vi "Dashboard Main.vi"() -> ()   [LabVIEW 2013]
uses:
  <vilib>/event_ctls.llb/eventvkey.ctl
  <vilib>/Rock Robotics/WPI/Dashboard/WPI_DashboardLogging Global.vi
  <vilib>/Utility/config.llb/Write Key (String).vi
  <vilib>/Utility/config.llb/Write Key (I32).vi
  <vilib>/Utility/config.llb/NI_LVConfig.lvlib
panel:
  in  "Camera Settings":T1={"Frame Rate"=30, "Compression"=30, "Size"=1} {"Frame Rate" scale=1.0..30.0; "Size" items=["640x480", "320x240", "160x120"]}
  out "fps":dbl format="%#.1g"
  out "Mbps":dbl format="%#.1g"
  out "Mbps 2":bool
  in  "DB Camera Config":bool
  out "Image Message":string="Timeout in Camera Communications"
  in  "Rec Mode":enum32{"Stop", "Record", "Playback"}(radio)
  in  "Dashboard Tab":T2(tab)
  out "Robot Mode":dbl
  out "Motor Current":dbl[](array[numeric])
  out "Compressor Relay Status":bool
  out "Compressor Control Status":bool
  in  "Compressor Control":bool
  in  "Jag Position Enable":bool
  out "Right Direction Motor Position":dbl
  out "Left Direction Motor Position":dbl
  out "MotorSliders R":cluster{"MotorSlide1":dbl, "MotorSlide2":dbl} {"MotorSlide2" scale=-1.0..1.0 scale format="%#_2e"; "MotorSlide1" scale=-1.0..1.0 scale format="%#_2e"}
  out "MotorChart R":cluster{"Numeric":dbl, "Numeric":dbl}(graph)
  out "MotorSliders L":T3 {"MotorSlide4 2" scale=0.0..14.0 scale format="%#_2e"; "MotorSlide2" scale=-1.0..1.0 scale format="%#_2e"; "MotorSlide1" scale=-1.0..1.0 scale format="%#_2e"}
  out "MotorChart L":T4(graph)
  out "JS1 Z":dbl(slide) scale=-1.0..1.0 scale format="%#_2e"
  out "Joystick 1":cluster{"X":dbl, "Y":dbl}[](graph)
  out "JS Buttons 1":T5
  out "JS2 Z":dbl(slide) scale=-1.0..1.0 scale format="%#_2e"
  out "Joystick 2":cluster{"X":dbl, "Y":dbl}[](graph)
  out "JS Buttons 2":T5
  out "Mode":T6(ring)=enum."Auto Disabled"
  out "Camera IP":string
  out "Jag 6":dbl(graph)
  out "Jag 1":dbl(graph)
  out "Jag 8":dbl(graph)
  out "Jag 3":dbl(graph)
  in  "Test Slider":dbl(slide) scale=0.0..100.0 scale format="%#_3g"
  in  "On/Off":bool caption="Solenoid"
  in  "Test Name":u16(ring) items=["Select the test to run..."]
  in  "Test Tree":string(tree)
  in  "Motor":cluster{"Value":dbl, "Enable":bool} {"Value" scale=-1.0..1.0 scale format="%#_3g"}
  out "Progress":T7 {"Test Progress" scale=0.0..100.0}
  in  "Rev/Fwd":cluster{"Forward":bool, "Reverse":bool}
  in  "Test Ring":u16(ring) items=["Auto", "Fixed indoor", "Fixed outdoor 1", "Fixed outdoor 2", "Fixed fluorescent 1", "Fixed fluorescent 2", "Hold current"]
  in  "Listbox":i32(listbox)
  out "Tree":string(tree)
  out "Camera Image":T8(plugin-control)
  in  "Enable":bool
  # "Left"
  # "Right"
  # "Battery"
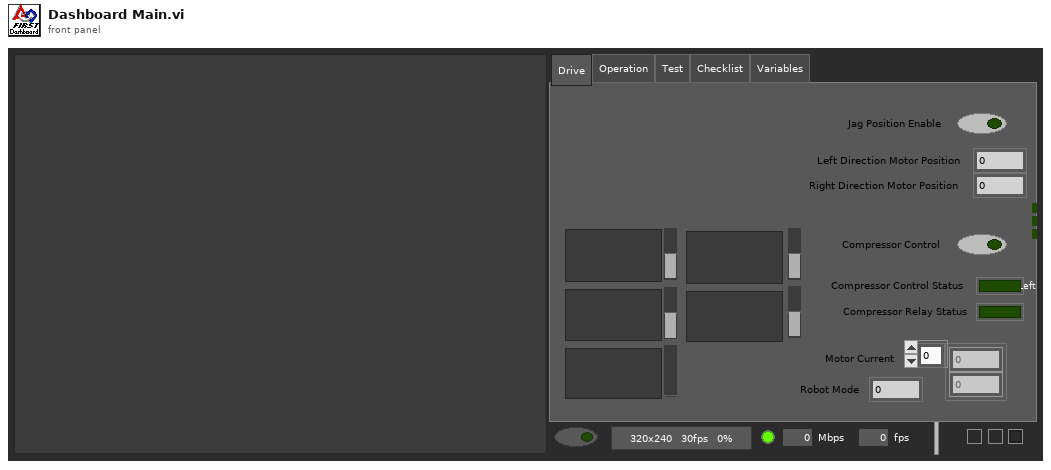
[diagram p1: front panel]
types:
  T1 = cluster{"Frame Rate":i32, "Compression":i32, "Size":u16}
  T2 = enum32{"Drive", "Operation", "Test", "Checklist", "Variables"}
  T3 = cluster{"MotorSlide1":dbl, "MotorSlide2":dbl, "MotorSlide4 2":dbl}
  T4 = cluster{"Numeric":dbl, "Numeric":dbl, "Battery":sgl}
  T5 = cluster{bool, bool, bool, bool, bool, bool, bool, bool, bool, bool, bool, bool}
  T6 = enum8{"Tele-Op Disabled", "Tele-Op Enabled", "Auto Disabled", "Auto Enabled", "Test Disabled", "Test Enabled", ""}
  T7 = cluster{"Test Progress":u8, "Test Progress Text":string}
  T8 = typedef "IMAQ Image.ctl" = refnum<image>
  T9 = enum32{"Drive", "Operation", "Auto", "Test", "Checklist", "Variables"}
  T10 = typedef "Image Type" = u32
  T11 = cluster{"Digital Inputs":bool[], "Digital Outputs":bool[]}
  T12 = cluster{"Competition mode":bool, "Robot Link":bool, "Autonomous":bool, "Enabled":bool, "E-Stop":bool, "Simulated":bool, "TestMode":bool, "Docked Window":bool}
  T13 = cluster{"Boolean Array[0]":bool, "Boolean Array[1]":bool, "Boolean Array[2]":bool, "Boolean Array[3]":bool, "Boolean Array[4]":bool, "Boolean Array[5]":bool, "Boolean Array[6]":bool, "Boolean Array[7]":bool, "Boolean Array[8]":bool, "Boolean Array[9]":bool, "Boolean Array[10]":bool, "Boolean Array[11]":bool}
  T14 = typedef "NI_LVConfig.lvlib/Config Data RefNum.ctl" = refnum<k1>
  T15 = typedef "eventvkey.ctl" = enum16{"ASCII", "Enter", "Return", "Shift", "Ctrl", "Alt", "Cmd", "Opt", "Caps", "NumLock", "Clear", "Break", "Up", "Down", "Left", "Right", "Insert", "Delete", "Home", "End", "PageUp", "PageDown", "Escape", "Help", "Pause", "ScrollLock", "F1", "F2", "F3", "F4", "F5", "F6", "F7", "F8", "F9", "F10", "F11", "F12", "F13", "F14", "F15", "F16", "F17", "F18", "F19", "F20", "F21", "F22", "F23", "F24", "Play", "VolumeUp", "VolumeDown", "Mute", "Two Byte Char"}
  T16 = cluster{"Image Size":bool, "Image Type":bool, "Pixel Value":bool, "ROI Information":bool, "Zoom Factor":bool}
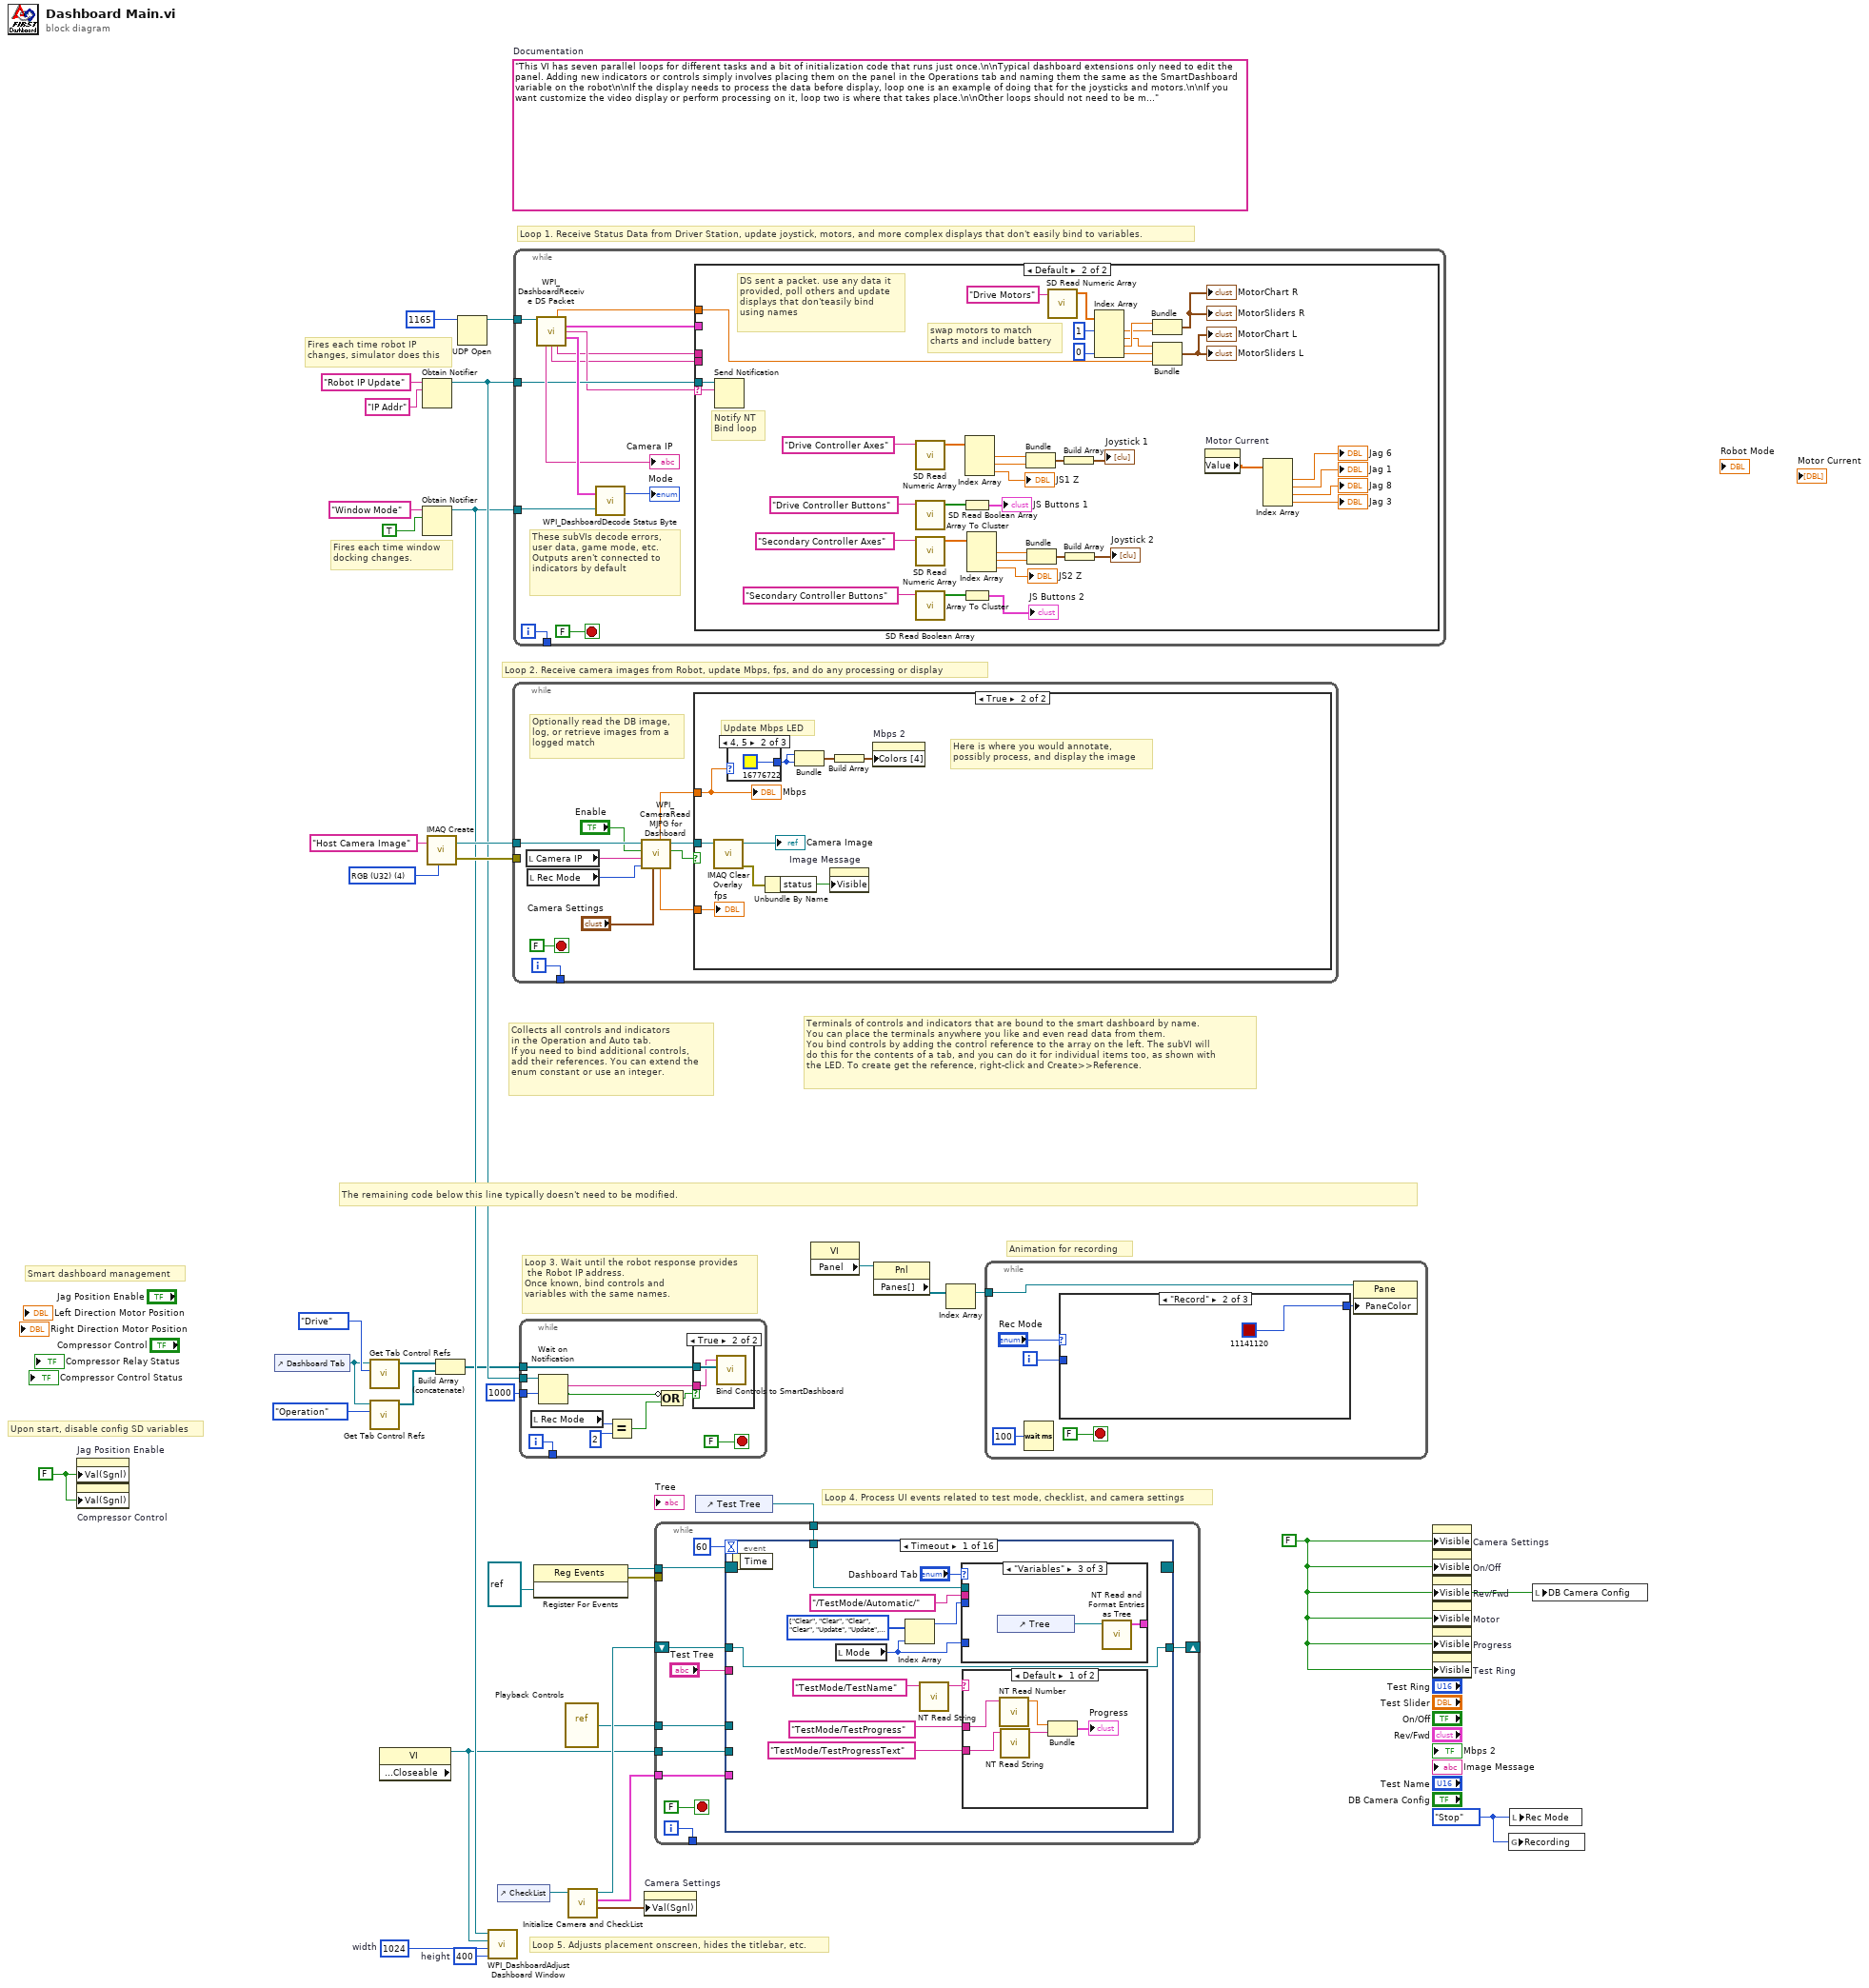
[diagram p0: block diagram]
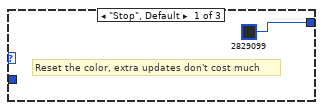
[diagram p2: hidden frame]
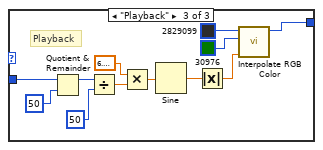
[diagram p3: hidden frame]
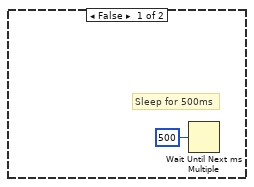
[diagram p5: hidden frame]
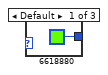
[diagram p6: hidden frame]
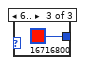
[diagram p7: hidden frame]
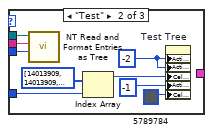
[diagram p9: hidden frame]
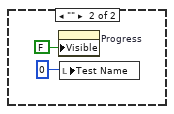
[diagram p10: hidden frame]
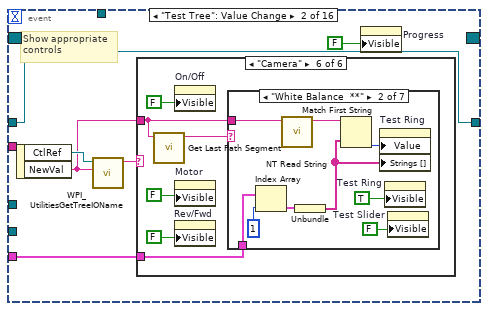
[diagram p11: hidden frame]
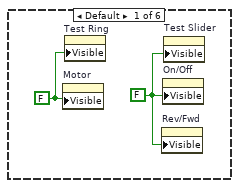
[diagram p12: hidden frame]
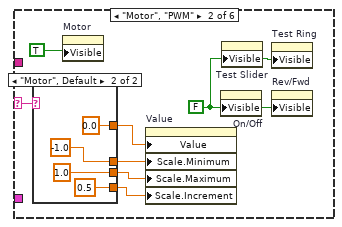
[diagram p13: hidden frame]
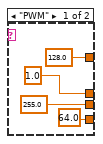
[diagram p14: hidden frame]
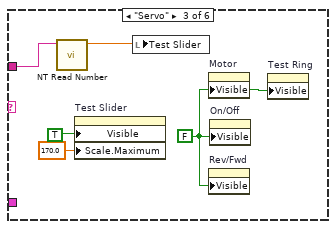
[diagram p15: hidden frame]
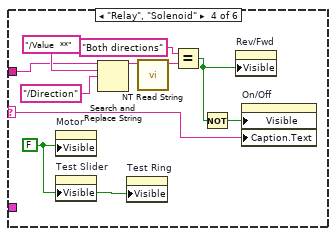
[diagram p16: hidden frame]
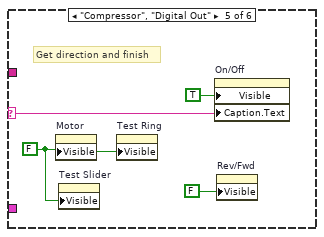
[diagram p17: hidden frame]
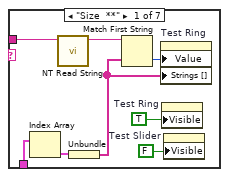
[diagram p18: hidden frame]
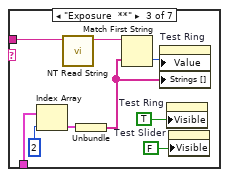
[diagram p19: hidden frame]
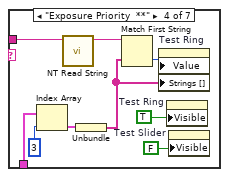
[diagram p20: hidden frame]
diagram:
  w1 = FALSE ("Value (Signaling)")
  w8 = enum32{"Stop", "Record", "Playback"}."Stop" ("Rec Mode")
  w11 = 400  # height
  w12 = 1024  # width
  w25 = FALSE ("Visible")
  (unwired) "This VI has seven parallel loops for different tasks and a bit of initialization code that runs just once.\n\nTypical dashboard extensions only need to edit the panel. Adding new indicators or controls simply involves placing them on the panel in the Operations tab and naming them the same as the SmartDashboard variable on the robot\n\nIf the display needs to process the data before display, loop one is an example of doing that for the joysticks and motors.\n\nIf you want customize the video display or perform processing on it, loop two is where that takes place.\n\nOther loops should not need to be modified. They are pretty standard, and document the task they perform."  # Documentation
  w35 = T10 4 items=["Grayscale (U8)", "Grayscale (I16)", "Grayscale (SGL)", "Complex (CSG)", "RGB (U32)", "HSL (U32)", "RGB (U64)"] ("Image Type")
  # "Upon start, disable config SD variables"
  # "Smart dashboard management"
  # "Animation for recording"
  # "Fires each time robot IP\nchanges, simulator does this"
  # "Fires each time window\ndocking changes."
  # "Collects all controls and indicators\nin the Operation and Auto tab.\nIf you need to bind additional controls,\nadd their references. You can extend the\nenum constant or use an integer."
  # "The remaining code below this line typically doesn't need to be modified."
  # "Loop 4. Process UI events related to test mode, checklist, and camera settings"
  # "Terminals of controls and indicators that are bound to the smart dashboard by name.\nYou can place the terminals anywhere you like and even read data from them.\nYou bind controls by adding the control reference to the array on the left. The subVI will\ndo this for the contents of a tab, and you can do it for individual items too, as shown with\nthe LED. To create get the reference, right-click and Create>>Reference."
  # "Loop 3. Wait until the robot response provides\n the Robot IP address.\nOnce known, bind controls and\nvariables with the same names."
  # "Loop 5. Adjusts placement onscreen, hides the titlebar, etc."
  # "Loop 1. Receive Status Data from Driver Station, update joystick, motors, and more complex displays that don't easily bind to variables."
  # "Loop 2. Receive camera images from Robot, update Mbps, fps, and do any processing or display"
  n1 = property on="Jag Position Enable" class="Bool (strict)"("Val(Sgnl)"=w1) -> ()  [unwired: 2 in, 2 out]
  n2 = property on="Compressor Control" class="Bool (strict)"("Val(Sgnl)"=w1) -> ()  [unwired: 2 in, 2 out]
  n3 = control-ref of="Dashboard Tab"() -> (w6:refnum<vi>)
  n4 = call <vilib>:"Get Tab Control Refs.vi"("Page Index"=T9."Drive" ("Dashboard Tab"), "TabControl in"=w6) -> ("ControlsOnPage"=w4:refnum<vi>[])  [unwired: 9 in]
  n5 = call <vilib>:"Get Tab Control Refs.vi"("Page Index"=T9."Operation" ("Dashboard Tab"), "TabControl in"=w6) -> ("ControlsOnPage"=w5:refnum<vi>[])  [unwired: 9 in]
  n6 = property class="VI" props=["Front Panel.Closeable"]() -> (reference out=w7:refnum<vi>)  [unwired: 2 in, 2 out]
  n7 = Obtain Notifier(name (unnamed)="Robot IP Update", notification data type="IP Addr" ("name (unnamed)")) -> (notifier out=w29:refnum<notifier>)  [unwired: 2 in, 2 out]
  n8 = Obtain Notifier(name (unnamed)="Window Mode", notification data type=TRUE) -> (notifier out=w10:refnum<notifier>)  [unwired: 2 in, 2 out]
  n9 = call "IMAQ Create"("Image Name"="Host Camera Image", "Image Type"=w35) -> ("New Image"=w33:T8, "error out"=w32:errorcluster)  [unwired: 2 in, 1 out]
  n10 = Build Array (concatenate)(w4, w5) -> (w3:refnum<vi>[])
  n11 = UDP Open(11:u16 1165 ("port")) -> (port=w36:refnum<k16>)  [unwired: 2 in, 4 out]
  n12 = call <vilib>:"WPI_DashboardAdjust Dashboard Window.vi"("height"=w11, "width"=w12, "reference in"=w7, "Notifier in"=w10) -> ()  [unwired: 8 in]
  n13 = control-ref of="CheckList"() -> (w9:refnum<vi>)
  n14 = while {
    tunnel: w33 -> [w46]
    tunnel: w32 -> [_]
    tunnel: [w47] -> _
    i -> [w47]
    stop <- FALSE stop-if-true
    # "Optionally read the DB image,\nlog, or retrieve images from a\nlogged match"
    n15 = local read "Camera IP"() -> (w39:string)
    n16 = local read "Rec Mode"() -> (w38:enum32{"Stop", "Record", "Playback"})
    n17 = call <vilib>:"WPI_CameraRead MJPG for Dashboard.vi"("Camera Settings"="Camera Settings", "Rec Mode"=w38, "Camera IP"=w39, "Enable"="Enable", "Refnum in"=w46) -> ("Active"=w43:bool, "Refnum out"=w45:T8, "FPS"=w42:dbl, "Bandwidth (Mbps)"=w41:dbl)  [unwired: 3 in]
    n18 = case shown="True" w43 {
      tunnel: w45 -> [_ w53]
      tunnel: w41 -> [_ w52]
      tunnel: w42 -> [_ w50]
      frame False {
        # "Sleep for 500ms"
        n19 = Wait Until Next ms Multiple(millisecond multiple=u32 500) -> ()  [unwired: 1 out]
      }
      frame True {
        # "Here is where you would annotate,\npossibly process, and display the image"
        # "Update Mbps LED"
        n20 = call "IMAQ Clear Overlay"("Image"=w53) -> ("error out"=w57:errorcluster, "Image Out"=→"Camera Image":T8)  [unwired: 2 in, 7 out]
        n21 = case shown="4, 5" w52 {
          tunnel: [u32 6618880 ("Color Box") u32 16776722 ("Color Box") u32 16716800 ("Color Box")] -> w54
          frame Default {
          }
          frame 4, 5 {
          }
          frame 6.. {
          }
        }
        n22 = Unbundle By Name(w57) -> ("status"=w58:bool)
        n23 = Bundle("Color Box"=w54, "Color Box"=w54) -> (w56:cluster{"Color Box":u32, "Color Box":u32})  [unwired: 1 out]
        n24 = property on="Image Message" class="Str"("Visible"=w58) -> ()  [unwired: 2 in, 2 out]
        n25 = Build Array(w56) -> (w55:cluster{"Color Box":u32, "Color Box":u32}[])
        n26 = property on="Mbps 2" class="Bool (strict)"("Colors [4]"=w55) -> ()  [unwired: 2 in, 2 out]
        "Mbps" <- w52
        "fps" <- w50
      }
    }
  }
  n27 = while {
    tunnel: w36 -> [w72]
    tunnel: w29 -> [w67]
    tunnel: w10 -> [w71]
    tunnel: [w68] -> _
    i -> [w68]
    stop <- FALSE stop-if-true
    # "These subVIs decode errors, user data, game mode, etc.\nOutputs aren't connected to indicators by default"
    n28 = call <vilib>:"WPI_DashboardReceive DS Packet.vi"("Recv Socket"=w72) -> ("Battery"=w62:sgl, "Driver Station"=w63:T11, "Robot IP Address"=w66:string, "Status"=w73:T12, "Camera IP Address"=→"Camera IP":string, "Low Priority User Data"=w65:string, "High Priority User Data"=w64:string)  [unwired: 1 in, 7 out]
    n29 = call <vilib>:"WPI_DashboardDecode Status Byte.vi"("Window Mode Notifier"=w71, "Status"=w73) -> ("Mode"=→"Mode":T6)  [unwired: 1 out]
    n30 = case shown="Default" w66 {
      selector: w66 -> [_ w90]
      tunnel: w67 -> [_ w91]
      tunnel: w65 -> [_ _]
      tunnel: w64 -> [_ _]
      tunnel: w63 -> [_ _]
      tunnel: w62 -> [_ w89]
      frame "0.0.0.0" {
        # "DS not sending packets, or no robot exists yet.\nDon't poll the variables"
      }
      frame Default {
        # "Notify NT\nBind loop"
        # "DS sent a packet. use any data it\nprovided, poll others and update\ndisplays that don'teasily bind\nusing names"
        # "swap motors to match\ncharts and include battery"
        n31 = Send Notification(notification=w90, notifier=w91) -> ()  [unwired: 1 in, 2 out]
        n32 = call <vilib>:"SD Read Numeric Array.vi"("Name"="Drive Controller Axes") -> ("Numeric Array"=w107:dbl[])  [unwired: 8 in, 2 out]
        n33 = call <vilib>:"SD Read Boolean Array.vi"("Name"="Drive Controller Buttons") -> ("Boolean Array"=w109:bool[])  [unwired: 8 in, 2 out]
        n34 = call <vilib>:"SD Read Numeric Array.vi"("Name"="Secondary Controller Axes") -> ("Numeric Array"=w101:dbl[])  [unwired: 8 in, 2 out]
        n35 = call <vilib>:"SD Read Boolean Array.vi"("Name"="Secondary Controller Buttons") -> ("Boolean Array"=w100:bool[])  [unwired: 8 in, 2 out]
        n36 = Array To Cluster(array=w109) -> (cluster=→"JS Buttons 1":T13)
        n37 = Array To Cluster(array=w100) -> (cluster=→"JS Buttons 2":T13)
        n38 = Index Array(array=w107) -> (element #1=w104:dbl, element #2=w105:dbl, element #3=→"JS1 Z":dbl)  [unwired: 3 in]
        n39 = Index Array(array=w101) -> (element #1=w96:dbl, element #2=w95:dbl, element #3=→"JS2 Z":dbl)  [unwired: 3 in]
        n40 = Bundle("Numeric"=w104, "Numeric"=w105) -> (w103:cluster{"Numeric":dbl, "Numeric":dbl})  [unwired: 1 in]
        n41 = Bundle("Numeric"=w96, "Numeric"=w95) -> (w97:cluster{"Numeric":dbl, "Numeric":dbl})  [unwired: 1 in]
        n42 = call <vilib>:"SD Read Numeric Array.vi"("Name"="Drive Motors") -> ("Numeric Array"=w88:dbl[])  [unwired: 8 in, 2 out]
        n43 = Build Array(w103) -> (→"Joystick 1":cluster{"Numeric":dbl, "Numeric":dbl}[])
        n44 = Build Array(w97) -> (→"Joystick 2":cluster{"Numeric":dbl, "Numeric":dbl}[])
        n45 = Index Array(array=w88, index #1=1, index #4=0) -> (element #1=w84:dbl, element #2=w83:dbl, element #3=w85:dbl, element #4=w80:dbl)  [unwired: 2 in]
        n46 = Bundle("Numeric"=w85, "Numeric"=w84) -> (→"MotorChart R" →"MotorSliders R":cluster{"Numeric":dbl, "Numeric":dbl})  [unwired: 1 in]
        n47 = Bundle("Numeric"=w83, "Numeric"=w80, "Battery"=w89) -> (→"MotorChart L" →"MotorSliders L":T4)  [unwired: 1 in]
        n48 = property on="Motor Current" class="Arr (strict)"() -> ("Value"=w75:dbl[])  [unwired: 2 in, 2 out]
        n49 = Index Array(array=w75) -> (element #1=→"Jag 6":dbl, element #2=→"Jag 1":dbl, element #3=→"Jag 8":dbl, element #4=→"Jag 3":dbl)  [unwired: 4 in]
      }
    }
  }
  n50 = while {
    tunnel: w3 -> [w123]
    tunnel: w29 -> [w121]
    tunnel: [w119] -> _
    tunnel: u32 1000 ("milliseconds to wait") -> [w118]
    i -> [w119]
    stop <- FALSE stop-if-true
    n51 = local read "Rec Mode"() -> (w114:enum32{"Stop", "Record", "Playback"})
    n52 = Wait on Notification(notifier=w121, timeout in ms (-1)=w118) -> (notification=w120:string, timed out?=w116:bool)  [unwired: 2 in, 2 out]
    n53 = Equal?(x=w114, y=u16 2 ("Rec Mode")) -> (x = y?=w115:bool)
    n54 = Compound Arithmetic op=OR(invert w116, w115) -> (w117:bool)
    n55 = case shown="True" w117 {
      tunnel: w123 -> [_ w125]
      tunnel: w120 -> [_ w124]
      frame False {
      }
      frame True {
        n56 = call <vilib>:"Bind Controls to SmartDashboard.vi"("Bound Control Refs"=w125, "Server IP Address"=w124) -> ()  [unwired: 10 in]
      }
    }
  }
  n57 = register-events(refnum<vi> refnum) -> (reference out=w16:refnum<event-registration>, error out=w15:errorcluster)  [unwired: 2 in]
  n58 = vi-ref "Playback Controls.vi"() -> (w17:refnum<vi>)
  n59 = call "Initialize Camera and CheckList.vi"("ListBox in"=w9) -> ("Cluster"=w23:cluster{"value":i32, "value":i32, "index":i32}, "Array"=w24:cluster{string[]}[], "File Refnum"=w22:T14)  [unwired: 8 in]
  n60 = property on="Camera Settings" class="Clust (strict)"("Val(Sgnl)"=w23) -> ()  [unwired: 2 in, 2 out]
  n61 = control-ref of="Test Tree"() -> (w21:refnum<vi>)
  n62 = while {
    tunnel: w24 -> [w133]
    shift-right: [w132] -> _
    shift-left: w22 -> [w131]
    tunnel: [w130] -> _
    tunnel: w21 -> [w129]
    tunnel: w17 -> [w128]
    tunnel: w16 -> [w127]
    tunnel: w15 -> [_]
    tunnel: w7 -> [w126]
    i -> [w130]
    stop <- FALSE stop-if-true
    n63 = event shown="[0] Timeout" {
      selector: w127 -> [_ _ _ _ _ _ _ _ _ _ _ _ _ _ _ _]
      dyn-events: [_ _ _ _ _ _ _ _ _ _ _ _ _ w371 _ _] -> _
      timeout: u32 60 ("milliseconds to wait") -> [_ _ _ _ _ _ _ _ _ _ _ _ _ _ _ _]
      tunnel: w129 -> [w143 _ _ _ _ _ _ _ _ _ _ _ _ _ _ _]
      tunnel: "Test Tree" -> [_ _ _ _ _ _ _ _ w340 w348 w350 w354 w362 _ _ _]
      tunnel: w133 -> [_ w167 _ _ _ _ w304 w334 _ _ _ _ _ _ _ _]
      tunnel: [w137 w166 w265 w270 w278 w290 w303 w327 w339 w346 w349 w353 w361 w373 w387 w388] -> w132
      tunnel: w131 -> [w137 w166 w265 w270 w278 w290 w302 w327 w339 w346 w349 w353 w361 w373 w387 w388]
      tunnel: w128 -> [_ _ _ _ _ _ _ _ _ _ _ _ _ w374 _ w391]
      tunnel: w126 -> [_ _ _ _ _ _ _ _ _ _ _ _ _ w369 _ _]
      event Timeout {
        w142 = enum16{"Update", "Clear"}[] [enum."Clear", enum."Clear", enum."Clear", enum."Clear", enum."Update", enum."Update", enum."Clear"] items=["Update", "Clear"]
        n64 = event-data() -> ()  [unwired: 1 in, 1 out]
        n65 = local read "Mode"() -> (w140:T6)
        n66 = Index Array(array=w142, index=w140) -> (element=w141:enum16{"Update", "Clear"})
        n67 = call <vilib>:"NT Read String.vi"("Name"="TestMode/TestName") -> ("String"=w146:string)  [unwired: 9 in, 1 out]
        n68 = case shown="\"Variables\"" "Dashboard Tab" {
          tunnel: w143 -> [_ w156 _]
          tunnel: "/TestMode/Automatic/" ("Name Pattern") -> [_ w155 _]
          tunnel: w141 -> [_ w154 _]
          tunnel: w140 -> [_ w152 _]
          tunnel: [_ _ w158] -> _
          frame "Operation", Default {
          }
          frame "Test" {
            w151 = -2 ("Active Item:Row Number")
            n69 = call <vilib>:"NT Read and Format Entries as Tree.vi"("Operation"=w154, "Name Pattern"=w155, "Tree Refnum"=w156) -> ()  [unwired: 7 in, 2 out]
            n70 = Index Array(array=u32[] [14013909, 14013909, 14013909, 14013909, 14013909, 16777215, 14013909], index=w152) -> (element=w150:u32)
            n71 = property on="Test Tree" class="Tree (strict)"("Active Item Row Number"=w151, "ActiveColNum"=w151, "CellBG"=w150, "Active Item Row Number"=-1 ("Active Item:Row Number"), "CellBG"=u32 5789784 ("Color Box")) -> ()  [unwired: 2 in, 2 out]
          }
          frame "Variables" {
            n72 = control-ref of="Tree"() -> (w157:refnum<vi>)
            n73 = call <vilib>:"NT Read and Format Entries as Tree.vi"("Tree Refnum"=w157) -> ("Formatted Strings"=w158:cluster{"Name":string, "Value":string}[])  [unwired: 9 in, 1 out]
          }
        }
        n74 = case shown="Default" w146 {
          tunnel: "TestMode/TestProgress" ("Name") -> [w160 _]
          tunnel: "TestMode/TestProgressText" ("Name") -> [w159 _]
          frame Default {
            n75 = call <vilib>:"NT Read Number.vi"("Name"=w160) -> ("Numeric"=w161:dbl)  [unwired: 9 in, 1 out]
            n76 = call <vilib>:"NT Read String.vi"("Name"=w159) -> ("String"=w162:string)  [unwired: 9 in, 1 out]
            n77 = Bundle("Numeric"=w161, "String"=w162) -> (→"Progress":cluster{"Numeric":dbl, "String":string})  [unwired: 1 in]
          }
          frame "" {
            n78 = property on="Progress" class="Clust (strict)"("Visible"=FALSE) -> ()  [unwired: 2 in, 2 out]
            n79 = local write "Test Name"(u16 0) -> ()
          }
        }
      }
      event "Test Tree": Value Change {
        # "Show appropriate\ncontrols"
        n80 = event-data() -> ("CtlRef"=w170:refnum<vi>, "NewVal"=w168:string)  [unwired: 1 in]
        n81 = call <vilib>:"WPI_UtilitiesGetTreeIOName.vi"("NewVal"=w168, "TreeControl in"=w170) -> ("I/O Name"=w171:string)  [unwired: 9 in]
        n82 = case shown="\"Camera\"" w171 {
          selector: w171 -> [_ w178 _ w196 w205 _]
          tunnel: w168 -> [_ _ w193 w195 _ w212]
          tunnel: w167 -> [_ _ _ _ _ w211]
          frame Default {
            w173 = FALSE ("Visible")
            w172 = FALSE ("Visible")
            n83 = property on="Motor" class="Clust (strict)"("Visible"=w172) -> ()  [unwired: 2 in, 2 out]
            n84 = property on="Test Ring" class="Ring (strict)"("Visible"=w172) -> ()  [unwired: 2 in, 2 out]
            n85 = property on="Rev/Fwd" class="Clust (strict)"("Visible"=w173) -> ()  [unwired: 2 in, 2 out]
            n86 = property on="On/Off" class="Bool (strict)"("Visible"=w173) -> ()  [unwired: 2 in, 2 out]
            n87 = property on="Test Slider" class="Slide (strict)"("Visible"=w173) -> ()  [unwired: 2 in, 2 out]
          }
          frame "Motor", "PWM" {
            w179 = FALSE ("Visible")
            n88 = case shown="\"Motor\", Default" w178 {
              tunnel: [1.0 ("Value") -1.0 ("Value")] -> w177
              tunnel: [255.0 ("Value") 1.0 ("Value")] -> w176
              tunnel: [128.0 ("Value") 0.0 ("Value")] -> w175
              tunnel: [64.0 ("Value") 0.5 ("Value")] -> w174
              frame "PWM" {
              }
              frame "Motor", Default {
              }
            }
            n89 = property on="Motor" class="Clust (strict)"("Visible"=TRUE) -> ()  [unwired: 2 in, 2 out]
            n90 = property on="Value" class="Slide (strict)"("Value"=w175, "Scale.Minimum"=w177, "Scale.Maximum"=w176, "Scale.Increment"=w174) -> ()  [unwired: 2 in, 2 out]
            n91 = property on="On/Off" class="Bool (strict)"("Visible"=w179) -> ()  [unwired: 2 in, 2 out]
            n92 = property on="Test Slider" class="Slide (strict)"("Visible"=w179) -> ()  [unwired: 2 in, 2 out]
            n93 = property on="Test Ring" class="Ring (strict)"("Visible"=w179) -> ()  [unwired: 2 in, 2 out]
            n94 = property on="Rev/Fwd" class="Clust (strict)"("Visible"=w179) -> ()  [unwired: 2 in, 2 out]
          }
          frame "Servo" {
            w191 = FALSE ("Visible")
            n95 = call <vilib>:"NT Read Number.vi"("Name"=w193) -> ("Numeric"=w192:dbl)  [unwired: 9 in, 1 out]
            n96 = property on="Test Slider" class="Slide (strict)"("Visible"=TRUE, "Scale.Maximum"=170.0 ("Scale.Range:Maximum")) -> ()  [unwired: 2 in, 2 out]
            n97 = local write "Test Slider"(w192) -> ()
            n98 = property on="Motor" class="Clust (strict)"("Visible"=w191) -> ()  [unwired: 2 in, 2 out]
            n99 = property on="Rev/Fwd" class="Clust (strict)"("Visible"=w191) -> ()  [unwired: 2 in, 2 out]
            n100 = property on="On/Off" class="Bool (strict)"("Visible"=w191) -> ()  [unwired: 2 in, 2 out]
            n101 = property on="Test Ring" class="Ring (strict)"("Visible"=w191) -> ()  [unwired: 2 in, 2 out]
          }
          frame "Relay", "Solenoid" {
            w194 = FALSE ("Visible")
            n102 = property on="Motor" class="Clust (strict)"("Visible"=w194) -> ()  [unwired: 2 in, 2 out]
            n103 = property on="Test Slider" class="Slide (strict)"("Visible"=w194) -> ()  [unwired: 2 in, 2 out]
            n104 = Search and Replace String(input string=w195, search string="/Value  **", replace string="/Direction") -> (result string=w201:string)  [unwired: 5 in, 3 out]
            n105 = property on="Test Ring" class="Ring (strict)"("Visible"=w194) -> ()  [unwired: 2 in, 2 out]
            n106 = call <vilib>:"NT Read String.vi"("Name"=w201) -> ("String"=w199:string)  [unwired: 9 in, 1 out]
            n107 = Equal?(x="Both directions", y=w199) -> (x = y?=w197:bool)
            n108 = Not(x=w197) -> (.not. x?=w198:bool)
            n109 = property on="Rev/Fwd" class="Clust (strict)"("Visible"=w197) -> ()  [unwired: 2 in, 2 out]
            n110 = property on="On/Off" class="Bool (strict)"("Visible"=w198, "Caption.Text"=w196) -> ()  [unwired: 2 in, 2 out]
          }
          frame "Compressor", "Digital Out" {
            w204 = FALSE ("Visible")
            # "Get direction and finish"
            n111 = property on="Motor" class="Clust (strict)"("Visible"=w204) -> ()  [unwired: 2 in, 2 out]
            n112 = property on="Test Slider" class="Slide (strict)"("Visible"=w204) -> ()  [unwired: 2 in, 2 out]
            n113 = property on="Test Ring" class="Ring (strict)"("Visible"=w204) -> ()  [unwired: 2 in, 2 out]
            n114 = property on="On/Off" class="Bool (strict)"("Visible"=TRUE, "Caption.Text"=w205) -> ()  [unwired: 2 in, 2 out]
            n115 = property on="Rev/Fwd" class="Clust (strict)"("Visible"=FALSE) -> ()  [unwired: 2 in, 2 out]
          }
          frame "Camera" {
            n116 = call <vilib>:"Get Last Path Segment.vi"("String in"=w212) -> ("String out"=w213:string)  [unwired: 10 in]
            n117 = property on="On/Off" class="Bool (strict)"("Visible"=FALSE) -> ()  [unwired: 2 in, 2 out]
            n118 = property on="Motor" class="Clust (strict)"("Visible"=FALSE) -> ()  [unwired: 2 in, 2 out]
            n119 = property on="Rev/Fwd" class="Clust (strict)"("Visible"=FALSE) -> ()  [unwired: 2 in, 2 out]
            n120 = case shown="\"White Balance  **\"" w213 {
              tunnel: w212 -> [w219 w228 w237 w246 w255 _ w261]
              tunnel: w211 -> [w217 w225 w234 w243 w252 _ _]
              frame "Size  **" {
                n121 = Index Array(array=w217) -> (element=w216:cluster{string[]})  [unwired: 1 in]
                n122 = call <vilib>:"NT Read String.vi"("Name"=w219) -> ("String"=w218:string)  [unwired: 9 in, 1 out]
                n123 = Unbundle(w216) -> (w214:string[])
                n124 = Match First String(2:w214, 3:w218) -> (0:w215:i32)  [unwired: 1 out]
                n125 = property on="Test Ring" class="Ring (strict)"("Value"=w215, "Strings []"=w214) -> ()  [unwired: 2 in, 2 out]
                n126 = property on="Test Ring" class="Ring (strict)"("Visible"=TRUE) -> ()  [unwired: 2 in, 2 out]
                n127 = property on="Test Slider" class="Slide (strict)"("Visible"=FALSE) -> ()  [unwired: 2 in, 2 out]
              }
              frame "White Balance  **" {
                n128 = Index Array(array=w225, index=1) -> (element=w226:cluster{string[]})
                n129 = call <vilib>:"NT Read String.vi"("Name"=w228) -> ("String"=w227:string)  [unwired: 9 in, 1 out]
                n130 = Unbundle(w226) -> (w223:string[])
                n131 = Match First String(2:w223, 3:w227) -> (0:w222:i32)  [unwired: 1 out]
                n132 = property on="Test Ring" class="Ring (strict)"("Value"=w222, "Strings []"=w223) -> ()  [unwired: 2 in, 2 out]
                n133 = property on="Test Ring" class="Ring (strict)"("Visible"=TRUE) -> ()  [unwired: 2 in, 2 out]
                n134 = property on="Test Slider" class="Slide (strict)"("Visible"=FALSE) -> ()  [unwired: 2 in, 2 out]
              }
              frame "Exposure  **" {
                n135 = Index Array(array=w234, index=2) -> (element=w235:cluster{string[]})
                n136 = call <vilib>:"NT Read String.vi"("Name"=w237) -> ("String"=w236:string)  [unwired: 9 in, 1 out]
                n137 = Unbundle(w235) -> (w231:string[])
                n138 = Match First String(2:w231, 3:w236) -> (0:w232:i32)  [unwired: 1 out]
                n139 = property on="Test Ring" class="Ring (strict)"("Value"=w232, "Strings []"=w231) -> ()  [unwired: 2 in, 2 out]
                n140 = property on="Test Ring" class="Ring (strict)"("Visible"=TRUE) -> ()  [unwired: 2 in, 2 out]
                n141 = property on="Test Slider" class="Slide (strict)"("Visible"=FALSE) -> ()  [unwired: 2 in, 2 out]
              }
              frame "Exposure Priority  **" {
                n142 = Index Array(array=w243, index=3) -> (element=w244:cluster{string[]})
                n143 = call <vilib>:"NT Read String.vi"("Name"=w246) -> ("String"=w245:string)  [unwired: 9 in, 1 out]
                n144 = Unbundle(w244) -> (w240:string[])
                n145 = Match First String(2:w240, 3:w245) -> (0:w241:i32)  [unwired: 1 out]
                n146 = property on="Test Ring" class="Ring (strict)"("Value"=w241, "Strings []"=w240) -> ()  [unwired: 2 in, 2 out]
                n147 = property on="Test Ring" class="Ring (strict)"("Visible"=TRUE) -> ()  [unwired: 2 in, 2 out]
                n148 = property on="Test Slider" class="Slide (strict)"("Visible"=FALSE) -> ()  [unwired: 2 in, 2 out]
              }
              frame "Color Enable  **" {
                n149 = Index Array(array=w252, index=4) -> (element=w253:cluster{string[]})
                n150 = call <vilib>:"NT Read String.vi"("Name"=w255) -> ("String"=w254:string)  [unwired: 9 in, 1 out]
                n151 = Unbundle(w253) -> (w249:string[])
                n152 = Match First String(2:w249, 3:w254) -> (0:w250:i32)  [unwired: 1 out]
                n153 = property on="Test Ring" class="Ring (strict)"("Value"=w250, "Strings []"=w249) -> ()  [unwired: 2 in, 2 out]
                n154 = property on="Test Ring" class="Ring (strict)"("Visible"=TRUE) -> ()  [unwired: 2 in, 2 out]
                n155 = property on="Test Slider" class="Slide (strict)"("Visible"=FALSE) -> ()  [unwired: 2 in, 2 out]
              }
              frame Default {
                n156 = property on="Test Ring" class="Ring (strict)"("Visible"=FALSE) -> ()  [unwired: 2 in, 2 out]
                n157 = property on="Test Slider" class="Slide (strict)"("Visible"=FALSE) -> ()  [unwired: 2 in, 2 out]
              }
              frame "Brightness  **", "Color Level  **", "Compression  **", "FPS  **", "Sharpness  **" {
                n158 = call <vilib>:"NT Read Number.vi"("Name"=w261) -> ("Numeric"=w260:dbl)  [unwired: 9 in, 1 out]
                n159 = local write "Test Slider"(w260) -> ()
                n160 = property on="Test Slider" class="Slide (strict)"("Visible"=TRUE, "Scale.Maximum"=100.0 ("Scale.Range:Maximum")) -> ()  [unwired: 2 in, 2 out]
                n161 = property on="Test Ring" class="Ring (strict)"("Visible"=FALSE) -> ()  [unwired: 2 in, 2 out]
              }
            }
          }
        }
        n162 = property on="Progress" class="Clust (strict)"("Visible"=FALSE) -> ()  [unwired: 2 in, 2 out]
      }
      event "Test Name": Mouse Enter {
        # "Populate the ring with the list of tests"
        n163 = event-data() -> ()  [unwired: 1 in, 1 out]
        n164 = call <vilib>:"NT Read String Array.vi"("Name"="TestMode/TestList") -> ("String Array"=w269:string[])  [unwired: 9 in, 1 out]
        n165 = Build Array (concatenate)("Select the test to run...", w269) -> (w268:string[])
        n166 = property on="Test Name" class="Ring (strict)"("Strings []"=w268) -> ()  [unwired: 2 in, 2 out]
      }
      event "Test Name": Value Change {
        w271 = FALSE ("Visible")
        # "Tell the robot the test name to run"
        n167 = event-data() -> ("NewVal"=w275:u16)  [unwired: 1 in]
        n168 = property on="Test Name" class="Ring (strict)"() -> ("Strings []"=w276:string[])  [unwired: 2 in, 2 out]
        n169 = local write "Progress"(T7 {"Test Progress"=0, "Test Progress Text"=""} ("Progress")) -> ()
        n170 = Index Array(array=w276, index=w275) -> (element=w274:string)
        n171 = call <vilib>:"NT Write String.vi"("String"=w274, "Name"="TestMode/TestName") -> ()  [unwired: 9 in, 1 out]
        n172 = property on="Progress" class="Clust (strict)"("Visible"=TRUE) -> ()  [unwired: 2 in, 2 out]
        n173 = property on="Motor" class="Clust (strict)"("Visible"=w271) -> ()  [unwired: 2 in, 2 out]
        n174 = property on="Test Slider" class="Slide (strict)"("Visible"=w271) -> ()  [unwired: 2 in, 2 out]
        n175 = property on="On/Off" class="Bool (strict)"("Visible"=w271) -> ()  [unwired: 2 in, 2 out]
        n176 = property on="Rev/Fwd" class="Clust (strict)"("Visible"=w271) -> ()  [unwired: 2 in, 2 out]
        n177 = property on="Test Ring" class="Ring (strict)"("Visible"=w271) -> ()  [unwired: 2 in, 2 out]
      }
      event "Listbox": Double Click {
        n178 = event-data() -> ("PlatMods.Shift"=w279:bool, "Row"=w281:i32)  [unwired: 1 in]
        n179 = case shown="True" w279 {
          tunnel: w281 -> [w285 _]
          tunnel: 1 -> [w284 _]
          frame False {
            n180 = property on="Listbox" class="LstBox (strict)"() -> ("Item Symbols"=w283:i32[])  [unwired: 2 in, 2 out]
            n181 = Replace Array Subset(array=w283, new element=w284, index=w285) -> (w282:i32[])
            n182 = property on="Listbox" class="LstBox (strict)"("Item Symbols"=w282) -> ()  [unwired: 2 in, 2 out]
          }
          frame True {
            w286 = 0 ("Top Row")
            n183 = property on="Listbox" class="LstBox (strict)"() -> ("Number of Rows"=w288:u32)  [unwired: 2 in, 2 out]
            n184 = Initialize Array(0, w288) -> (w287:i32[])
            n185 = property on="Listbox" class="LstBox (strict)"("Top Row"=w286, "Value"=w286, "Item Symbols"=w287) -> ()  [unwired: 2 in, 2 out]
          }
        }
      }
      event "Listbox": Key Down {
        n186 = event-data() -> ("VKey"=w292:T15)  [unwired: 1 in]
        n187 = case shown="\"Left\", \"Right\"" w292 {
          selector: w292 -> [w297 _]
          tunnel: eventvkey."Left" ("VKey") -> [w295 _]
          frame "Left", "Right" {
            n188 = Equal?(x=w295, y=w297) -> (x = y?=w296:bool)
            n189 = Select(t=0, s=w296, f=1) -> (s? t:f=w298:i32)
            n190 = property on="Listbox" class="LstBox (strict)"() -> ("Item Symbols"=w301:i32[])  [unwired: 2 in, 2 out]
            n191 = Replace Array Subset(array=w301, new element=w298, index="Listbox") -> (w300:i32[])
            n192 = property on="Listbox" class="LstBox (strict)"("Item Symbols"=w300) -> ()  [unwired: 2 in, 2 out]
          }
          frame Default {
          }
        }
      }
      event "DB Camera Config": Value Change {
        n193 = event-data() -> ("NewVal"=w305:bool)  [unwired: 1 in]
        n194 = case shown="False" w305 {
          tunnel: w304 -> [w314 _]
          tunnel: [w307 w325] -> w303
          tunnel: w302 -> [w306 w325]
          frame False {
            w321 = "Camera"
            w324 = FALSE ("Visible")
            n195 = local read "Camera Settings"() -> (w313:T1)
            n196 = Index Array(array=w314) -> (element=w317:cluster{string[]})  [unwired: 1 in]
            n197 = Unbundle(w313) -> ("Frame Rate"=w312:i32, "Compression"=w311:i32, "Size"=w315:u16)
            n198 = Unbundle(w317) -> (w316:string[])
            n199 = Index Array(array=w316, index=w315) -> (element=w310:string)
            n200 = call-poly <vilib>:"Write Key.vi"("section"=w321, "value"=w310, "key"="Size", "refnum"=w306) -> ("refnum out"=w323:T14)  [unwired: 2 in, 5 out]
            n201 = call-poly <vilib>:"Write Key.vi"("section"=w321, "value"=w312, "key"="FrameRate", "refnum"=w323) -> ("refnum out"=w322:T14)  [unwired: 1 in, 6 out]
            n202 = property on="Camera Settings" class="Clust (strict)"("Visible"=w324) -> ()  [unwired: 2 in, 2 out]
            n203 = local write "DB Camera Config"(w324) -> ()
            n204 = call-poly <vilib>:"Write Key.vi"("section"=w321, "value"=w311, "key"="Compression", "refnum"=w322) -> ("refnum out"=w308:T14)  [unwired: 1 in, 6 out]
            n205 = call <vilib>:"Close Config Data.vi"("refnum"=w308) -> ("file path"=w309:path)  [unwired: 2 in, 8 out]
            n206 = call <vilib>:"Open Config Data.vi"("configuration file path"=w309) -> ("refnum"=w307:T14)  [unwired: 8 in, 2 out]
          }
          frame True {
            n207 = property on="Camera Settings" class="Clust (strict)"("Visible"=TRUE) -> ()  [unwired: 2 in, 2 out]
          }
        }
      }
      event "Camera Settings": Value Change {
        n208 = event-data() -> ("NewVal"=w338:T1)  [unwired: 1 in]
        n209 = Index Array(array=w334) -> (element=w333:cluster{string[]})  [unwired: 1 in]
        n210 = Unbundle(w338) -> ("Frame Rate"=w329:i32, "Compression"=w328:i32, "Size"=w331:u16)
        n211 = Unbundle(w333) -> (w332:string[])
        n212 = Index Array(array=w332, index=w331) -> (element=w330:string)
        n213 = Format Into String(format string="%s   %dfps   %d%%", w330, w329, w328) -> (resulting string=w335:string)  [unwired: 2 in, 1 out]
        n214 = Build Array(w335) -> (w336:string[])
        n215 = property on="DB Camera Config" class="Bool (strict)"("Strings [4]"=w336) -> ()  [unwired: 2 in, 2 out]
      }
      event "Motor.Enable": Value Change {
        n216 = event-data() -> ("NewVal"=w344:bool)  [unwired: 1 in]
        n217 = Unbundle("Motor") -> ("Value"=w343:dbl)  [unwired: 1 out]
        n218 = Select(t=w343, s=w344, f=0.0) -> (s? t:f=w341:dbl)
        n219 = call <vilib>:"NT Write Number.vi"("Numeric"=w341, "Name"=w340) -> ()  [unwired: 9 in, 1 out]
      }
      event "Test Slider": Value Change {
        n220 = event-data() -> ("NewVal"=w347:dbl)  [unwired: 1 in]
        n221 = call <vilib>:"NT Write Number.vi"("Numeric"=w347, "Name"=w348) -> ()  [unwired: 9 in, 1 out]
      }
      event "On/Off": Value Change {
        n222 = event-data() -> ("NewVal"=w352:bool)  [unwired: 1 in]
        n223 = Boolean To (0,1)(Boolean=w352) -> (0, 1=w351:i16)
        n224 = call <vilib>:"NT Write Number.vi"("Numeric"=w351, "Name"=w350) -> ()  [unwired: 9 in, 1 out]
      }
      event "Rev/Fwd": Value Change {
        n225 = event-data() -> ("NewVal.Forward"=w360:bool, "NewVal.Reverse"=w359:bool)  [unwired: 1 in]
        n226 = Boolean To (0,1)(Boolean=w360) -> (0, 1=w356:i16)
        n227 = Boolean To (0,1)(Boolean=w359) -> (0, 1=w358:i16)
        n228 = Negate(x=w358) -> (-x=w357:i16)
        n229 = Add(x=w356, y=w357) -> (x+y=w355:i16)
        n230 = call <vilib>:"NT Write Number.vi"("Numeric"=w355, "Name"=w354) -> ()  [unwired: 9 in, 1 out]
      }
      event "Test Ring": Value Change {
        n231 = event-data() -> ("NewVal"=w364:u16)  [unwired: 1 in]
        n232 = property on="Test Ring" class="Ring (strict)"() -> ("Strings []"=w365:string[])  [unwired: 2 in, 2 out]
        n233 = Index Array(array=w365, index=w364) -> (element=w363:string)
        n234 = call <vilib>:"NT Write String.vi"("String"=w363, "Name"=w362) -> ()  [unwired: 9 in, 1 out]
      }
      event "Rec Mode": Value Change {
        # "Update globals for recording mode and path to read log from.\nClear when logging and let NetworkTables set path for vision to\nuse."
        n235 = event-data() -> ("NewVal"=w375:enum32{"Stop", "Record", "Playback"})  [unwired: 1 in]
        n236 = global write "WPI_DashboardLogging Global.vi" "Logging Filename"(path "") -> ()
        n237 = case shown="\"Stop\", \"Record\"" w375 {
          tunnel: w374 -> [_ w377 w385]
          tunnel: [_ _ w384] -> w371
          tunnel: [_ _ w383] -> _
          tunnel: w369 -> [_ _ w381]
          tunnel: cluster{i32, i32} {-250, 170} -> [_ _ w380]
          tunnel: [_ _ T16 {"Image Size"=TRUE, "Image Type"=TRUE, "Pixel Value"=TRUE, "ROI Information"=TRUE, "Zoom Factor"=FALSE} ("Image Information Shown:All Elements")] -> w367
          tunnel: [_ _ TRUE ("Zoom Factor")] -> w366
          frame Default {
          }
          frame "Stop", "Record" {
            # "Place Window too"
            n238 = invoke class="VI" method="FP.Close"(reference=w377) -> (reference out=w376:refnum<vi>)  [unwired: 2 in, 2 out]
            n239 = invoke class="VI" method="Abort VI"(reference=w376) -> ()  [unwired: 2 in, 3 out]
          }
          frame "Playback" {
            n240 = call "Open Playback Panel.vi"("Offset"=w380, "DB VI Ref"=w381, "Playback in"=w385) -> ("Playback out"=w382:refnum<vi>)  [unwired: 8 in]
            n241 = register-events(w382) -> (reference out=w384:refnum<event-registration>, error out=w383:errorcluster)  [unwired: 2 in]
          }
        }
        n242 = global write "WPI_DashboardLogging Global.vi" "Recording"(w375) -> ()
        n243 = property on="Camera Image" class="ImageControl"("Image Information Shown"=w367, "Image Information Visible"=w366) -> ()  [unwired: 2 in, 2 out]
        n244 = call <vilib>:"WPI_DashboardNT Log FieldName Cache.vi"("Operation"=enum16{"Lookup/Add", "Index", "Clear"}."Clear") -> ()  [unwired: 8 in, 3 out]
      }
      event Panel Close {
        w386 = enum32{"Stop", "Record", "Playback"}."Stop" ("Rec Mode")
        n245 = event-data() -> ()  [unwired: 1 in, 4 out]
        n246 = local write "Rec Mode"(w386) -> ()
        n247 = global write "WPI_DashboardLogging Global.vi" "Recording"(w386) -> ()
      }
      event Panel Close {
        # "Abort playback window and ourself"
        n248 = event-data() -> ()  [unwired: 1 in, 4 out]
        n249 = invoke class="VI" method="FP.Close"(reference=w391) -> (reference out=w390:refnum<vi>)  [unwired: 2 in, 2 out]
        n250 = invoke class="VI" method="Abort VI"(reference=w390) -> (error out=w389:errorcluster)  [unwired: 2 in, 2 out]
        n251 = invoke class="VI" method="Abort VI"(error in=w389) -> ()  [unwired: 2 in, 3 out]
      }
    }
  }
  n252 = property class="VI"() -> ("Panel"=w19:refnum<vi>)  [unwired: 2 in, 2 out]
  n253 = property class="Pnl"(reference=w19) -> ("Panes[]"=w20:refnum<vi>[])  [unwired: 1 in, 2 out]
  n254 = Index Array(array=w20) -> (element=w18:refnum<vi>)  [unwired: 1 in]
  n255 = while {
    tunnel: w18 -> [w393]
    i -> [w396]
    stop <- FALSE stop-if-true
    n256 = Wait (ms)(milliseconds to wait=u32 100) -> ()  [unwired: 1 out]
    n257 = case shown="\"Record\"" "Rec Mode" {
      tunnel: w396 -> [_ _ w411]
      tunnel: [u32 2829099 ("Base Color") u32 11141120 ("Target Color") w400] -> w392
      frame "Stop", Default {
        # "Reset the color, extra updates don't cost much"
      }
      frame "Record" {
      }
      frame "Playback" {
        # "Playback"
        n258 = Quotient & Remainder(x=w411, y=u32 50 ("milliseconds to wait")) -> (x-y*floor(x/y)=w407:u32)  [unwired: 1 out]
        n259 = Divide(x=w407, y=u32 50 ("milliseconds to wait")) -> (x/y=w404:dbl)
        n260 = Multiply(x=6.283185307179586, y=w404) -> (x*y=w409:dbl)
        n261 = Sine(x=w409) -> (sin(x)=w408:dbl)
        n262 = Absolute Value(x=w408) -> (abs(x)=w401:dbl)
        n263 = call "Interpolate RGB Color.vi"("Proportion"=w401, "Target Color"=u32 30976, "Base Color"=u32 2829099) -> ("Result Color"=w400:u32)  [unwired: 8 in]
      }
    }
    n264 = property class="Pane"(reference=w393, "PaneColor"=w392) -> ()  [unwired: 1 in, 2 out]
  }
  n265 = property on="Camera Settings" class="Clust (strict)"("Visible"=w25) -> ()  [unwired: 2 in, 2 out]
  n266 = property on="On/Off" class="Bool (strict)"("Visible"=w25) -> ()  [unwired: 2 in, 2 out]
  n267 = property on="Rev/Fwd" class="Clust (strict)"("Visible"=w25) -> ()  [unwired: 2 in, 2 out]
  n268 = property on="Motor" class="Clust (strict)"("Visible"=w25) -> ()  [unwired: 2 in, 2 out]
  n269 = property on="Progress" class="Clust (strict)"("Visible"=w25) -> ()  [unwired: 2 in, 2 out]
  n270 = property on="Test Ring" class="Ring (strict)"("Visible"=w25) -> ()  [unwired: 2 in, 2 out]
  n271 = global write "WPI_DashboardLogging Global.vi" "Recording"(w8) -> ()
  n272 = local write "Rec Mode"(w8) -> ()
  n273 = local write "DB Camera Config"(w25) -> ()
